vi "Downsample Timseries.vi"(10 "Factor":u32=3333, 11 "Waveform New":cluster{dbl, dbl, dbl[][]} {"?" format="%_8g"}) -> (3 "Waveform Downsampled":cluster{dbl, dbl, dbl[][]} {"?" format="%_8g"})   [LabVIEW 2020]
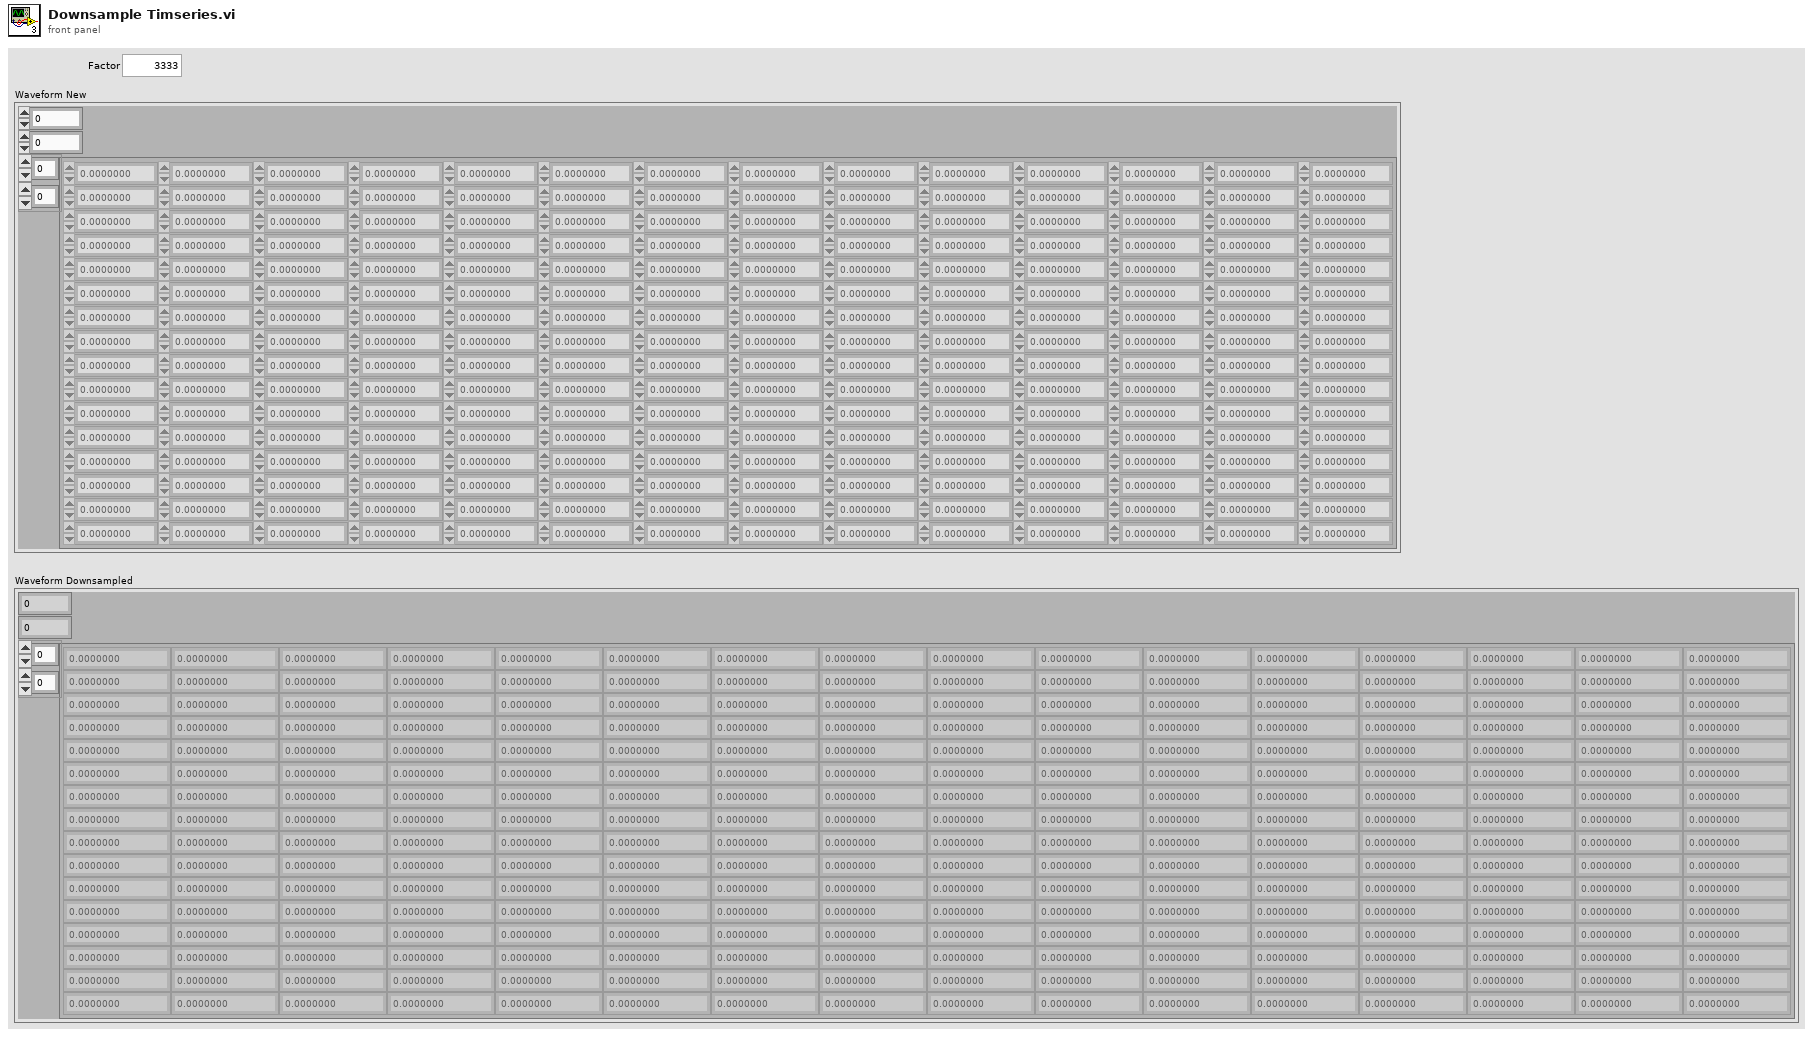
[diagram p1: front panel]
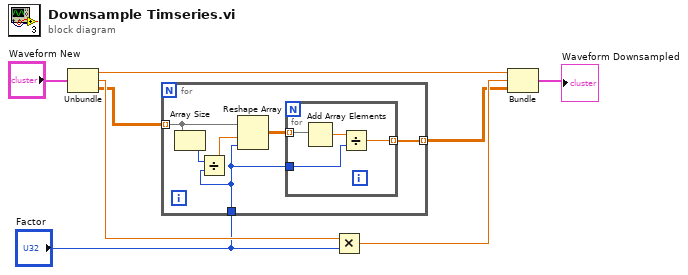
[diagram p0: block diagram]
diagram:
  n1 = Unbundle("Waveform New") -> (w4:dbl, w7:dbl, w2:dbl[][])
  n2 = for {
    tunnel: w2 -> [w9] mode=indexing
    tunnel: [w13] -> w1 mode=indexing
    tunnel: "Factor" -> [w11]
    n3 = Array Size(array=w9) -> (size(s)=w10:i32)
    n4 = Divide(x=w10, y=w11) -> (x/y=w12:dbl)
    n5 = Reshape Array(w9, w12, w11) -> (w14:dbl[][])
    n6 = for {
      tunnel: w14 -> [w18] mode=indexing
      tunnel: [w16] -> w13 mode=indexing
      tunnel: w11 -> [w15]
      n7 = Add Array Elements(numeric array=w18) -> (sum=w17:dbl)
      n8 = Divide(x=w17, y=w15) -> (x/y=w16:dbl)
    }
  }
  n9 = Multiply(x=w7, y="Factor") -> (x*y=w5:dbl)
  n10 = Bundle(w4, w5, w1) -> (→"Waveform Downsampled":cluster{dbl, dbl, dbl[][]})  [unwired: 1 in]
